vi "1.Log插入Subpanel.vi"(8 "Error In":errorcluster, 10 "Sub Panel":refnum<vi>, 11 "Module ID":i32=-1) -> (0 "error out":errorcluster, 3 "Module ID out":i32=-1)   [LabVIEW 2020, in "Log.lvlib"]
uses:
  Log.lvlib
  Log.lvlibp
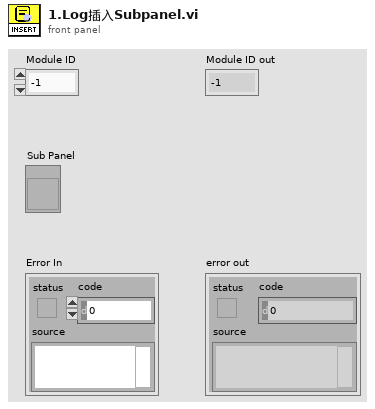
[diagram p1: front panel]
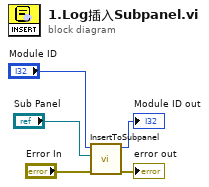
[diagram p0: block diagram]
diagram:
  n1 = call "InsertToSubpanel.vi"("Error In"="Error In", "Sub Panel"="Sub Panel", "Module ID"="Module ID") -> ("error out"=→"error out":errorcluster, "Module ID out"=→"Module ID out":i32)  [unwired: 7 in]
